vi "Move Left To Matrix.vi"(3 "Make Vertical":bool, 5 "Label":string="Test", 6 "Wait Time":dbl, 8 "error in":errorcluster, 9 "Speed (mm/s)":dbl=50.0, 10 "Offset":T1 format="%.3f", 11 "Location":string) -> (0 "error out":errorcluster)   [LabVIEW 2013]
uses:
  <vilib>/Analysis/Matrix/Datatypes/RealMatrix.ctl
  <vilib>/Analysis/Matrix/NI_Matrix.lvlib
panel:
  out "Final Offset":T1 format="%.3f"
  in  "Alt Goal":T2
  in  "Start":T1 format="%.3f"
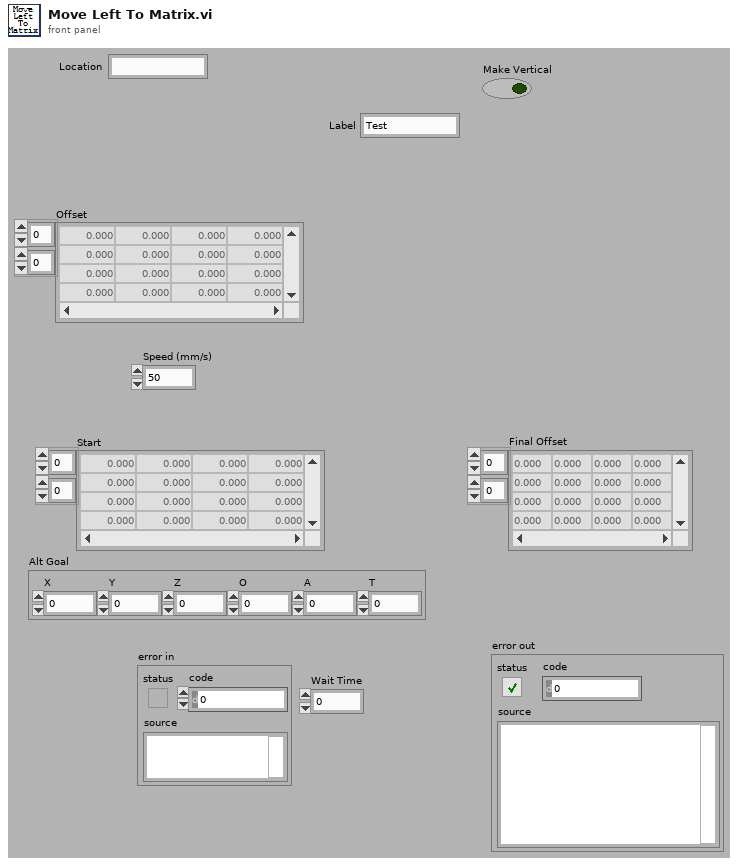
[diagram p1: front panel]
types:
  T1 = typedef "NI_Matrix.lvlib/RealMatrix.ctl" = dbl[][]
  T2 = cluster{"X":dbl, "Y":dbl, "Z":dbl, "O":dbl, "A":dbl, "T":dbl}
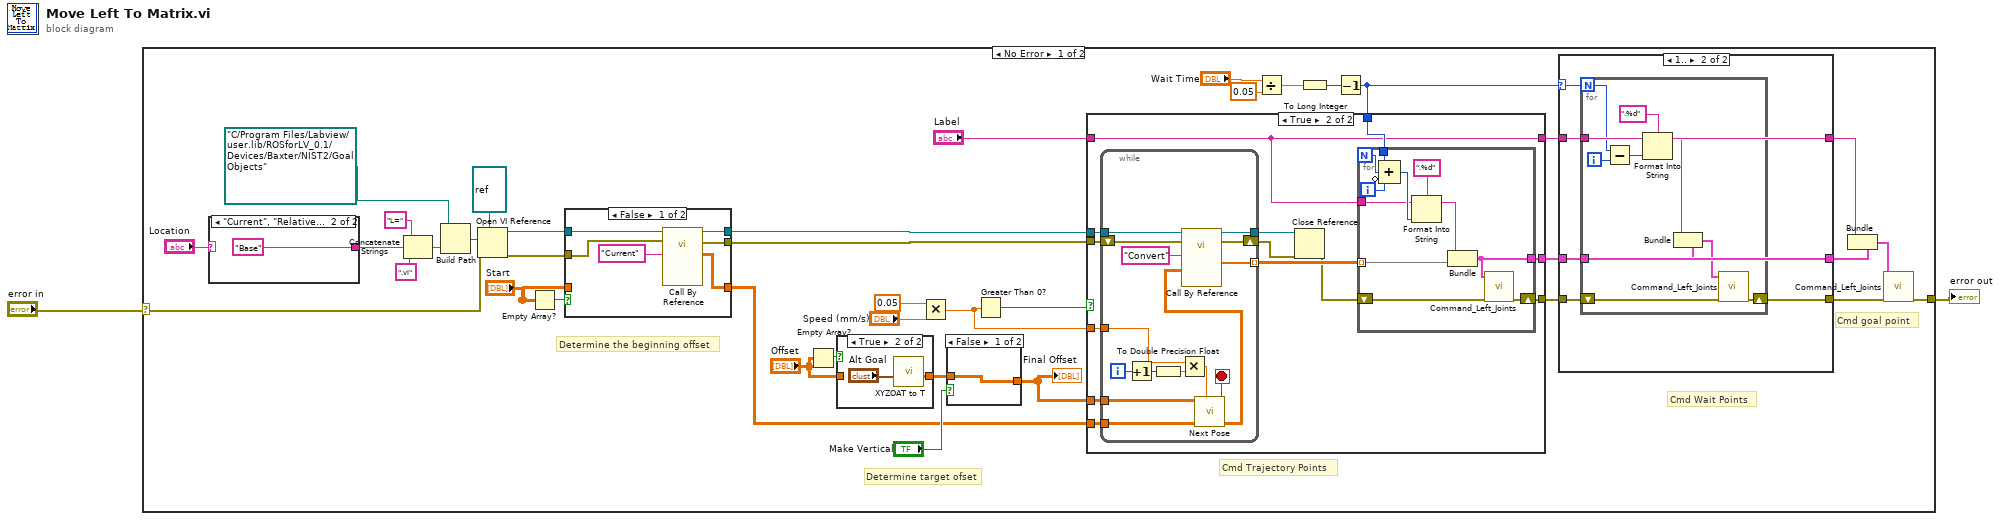
[diagram p0: block diagram]
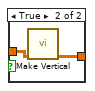
[diagram p5: hidden frame]
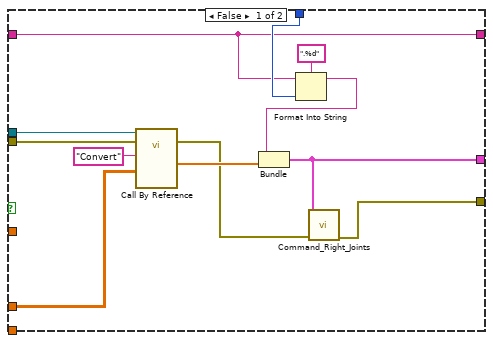
[diagram p6: hidden frame]
diagram:
  n1 = case shown="No Error" "error in" {
    selector: "error in" -> [w17 w128]
    tunnel: [w5 w128] -> w1
    frame No Error {
      # "Determine target ofset"
      # "Determine the beginning offset"
      # "Cmd goal point"
      # "Cmd Wait Points"
      # "Cmd Trajectory Points"
      n2 = case shown="\"Current\", \"Relative\"" "Location" {
        selector: "Location" -> [w51 _]
        tunnel: [w51 "Base"] -> w20
        frame Default {
        }
        frame "Current", "Relative" {
        }
      }
      n3 = Concatenate Strings("L=", w20, ".vi" ("string")) -> (w27:string)
      n4 = Build Path(base path=path "C:/Program Files/Labview/user.lib/ROSforLV_0.1/Devices/Baxter/NIST2/Goal Objects", name or relative path=w27) -> (appended path=w28:path)
      n5 = Open VI Reference(type specifier VI Refnum (for type only)=refnum<vi> refnum, vi path=w28, error in (no error)=w17) -> (vi reference=w25:refnum<vi>, error out=w26:errorcluster)  [unwired: 3 in]
      n6 = Empty Array?(array="Start") -> (empty?=w19:bool)
      n7 = case shown="False" w19 {
        tunnel: [w47 w48] -> w11
        tunnel: w26 -> [w46 w48]
        tunnel: [w45 w49] -> w12
        tunnel: w25 -> [w43 w49]
        tunnel: "Start" -> [_ w50]
        tunnel: [w42 w50] -> w16
        frame False {
          n8 = call-by-ref "?"(reference=w43, error in=w46, "Command"="Current") -> (reference out=w45:refnum<vi>, error out=w47:errorcluster, "Matrix"=w42:T1)  [unwired: 8 in, 2 out]
        }
        frame True {
        }
      }
      n9 = Empty Array?(array="Offset") -> (empty?=w41:bool)
      n10 = case shown="True" w41 {
        tunnel: "Offset" -> [w125 _]
        tunnel: [w125 w126] -> w37
        frame False {
        }
        frame True {
          n11 = call "XYZOAT to T.vi"("XYZOAT"="Alt Goal") -> ("T"=w126:T1)  [unwired: 10 in]
        }
      }
      n12 = Multiply(x=0.05 ("y"), y="Speed (mm/s)") -> (x*y=w13:dbl)
      n13 = case shown="False" "Make Vertical" {
        tunnel: w37 -> [w71 w73]
        tunnel: [w71 w72] -> w36
        frame False {
        }
        frame True {
          n14 = call "Make Vertical.vi"("Matrix"=w73) -> ("Vertical Matrix"=w72:T1)  [unwired: 10 in]
        }
      }
      "Final Offset" <- w36
      n15 = Greater Than 0?(x=w13) -> (x > 0?=w40:bool)
      n16 = Divide(x="Wait Time", y=0.05) -> (x/y=w31:dbl)
      n17 = To Long Integer(number=w31) -> (32bit integer=w30:i32)
      n18 = Decrement(x=w30) -> (x-1=w32:i32)
      n19 = case shown="True" w40 {
        tunnel: w16 -> [_ w98]
        tunnel: "Label" -> [w74 w89]
        tunnel: w36 -> [w82 w97]
        tunnel: w13 -> [_ w95]
        tunnel: w32 -> [w76 w96]
        tunnel: w12 -> [w84 w94]
        tunnel: w11 -> [w83 w93]
        tunnel: [w80 w91] -> w10
        tunnel: [w78 w90] -> w8
        tunnel: [w74 w89] -> w9
        frame False {
          n20 = call-by-ref "?"(reference=w84, error in=w83, "Matrix"=w82, "Command"="Convert") -> (error out=w79:errorcluster, "Joints"=w81:dbl[])  [unwired: 7 in, 3 out]
          n21 = Format Into String(format string=".%d", initial string=w74, w76) -> (resulting string=w75:string)  [unwired: 1 in, 1 out]
          n22 = Bundle(w75, "Joints"=w81) -> (w80:cluster{string, "Joints":dbl[]})  [unwired: 1 in]
          n23 = call "Command_Right_Joints.vi"("error in"=w79, "Goal"=w80) -> ("error out"=w78:errorcluster)  [unwired: 6 in, 1 out]
        }
        frame True {
          n24 = while {
            tunnel: w98 -> [w119]
            tunnel: w97 -> [w118]
            tunnel: w95 -> [w121]
            tunnel: w94 -> [w115]
            tunnel: [w112] -> w92 mode=indexing
            shift-right: [w111] -> w87
            shift-left: w93 -> [w114]
            tunnel: [w110] -> w88
            i -> [w123]
            stop <- w124 stop-if-true
            n25 = Increment(x=w123) -> (x+1=w117:i32)
            n26 = To Double Precision Float(number=w117) -> (double precision float=w122:dbl)
            n27 = Multiply(x=w121, y=w122) -> (x*y=w120:dbl)
            n28 = call "Next Pose.vi"("Step"=w120, "Start"=w119, "Goal"=w118) -> ("Pose"=w113:T1, "At Goal"=w124:bool)  [unwired: 7 in]
            n29 = call-by-ref "?"(reference=w115, error in=w114, "Matrix"=w113, "Command"="Convert") -> (reference out=w110:refnum<vi>, error out=w111:errorcluster, "Joints"=w112:dbl[])  [unwired: 7 in, 2 out]
          }
          n30 = Close Reference(reference=w88, error in (no error)=w87) -> (error out=w86:errorcluster)
          n31 = for {
            N -> [w109]
            tunnel: w89 -> [w105]
            tunnel: w96 -> [w104]
            tunnel: w92 -> [w102] mode=indexing
            shift-right: [w100] -> w90
            shift-left: w86 -> [w101]
            tunnel: [w99] -> w91
            i -> [w108]
            n32 = Compound Arithmetic op=ADD(w104, w109, invert w108) -> (w106:i32)
            n33 = Format Into String(format string=".%d", initial string=w105, w106) -> (resulting string=w103:string)  [unwired: 1 in, 1 out]
            n34 = Bundle(w103, "Joints"=w102) -> (w99:cluster{string, "Joints":dbl[]})  [unwired: 1 in]
            n35 = call "Command_Left_Joints.vi"("error in"=w101, "Goal"=w99) -> ("error out"=w100:errorcluster)  [unwired: 6 in, 1 out]
          }
        }
      }
      n36 = case shown="1.." w32 {
        selector: w32 -> [_ w60]
        tunnel: w10 -> [w54 w57]
        tunnel: w9 -> [w53 w56]
        tunnel: w8 -> [w55 w59]
        tunnel: [w55 w58] -> w4
        tunnel: [w54 w57] -> w7
        tunnel: [w53 w56] -> w6
        frame ..0 {
        }
        frame 1.. {
          n37 = for {
            N: w60 -> [w69]
            tunnel: w56 -> [w64]
            tunnel: w57 -> [w66]
            shift-right: [w63] -> w58
            shift-left: w59 -> [w62]
            i -> [w68]
            n38 = Subtract(x=w69, y=w68) -> (x-y=w70:i32)
            n39 = Format Into String(format string=".%d", initial string=w64, w70) -> (resulting string=w65:string)  [unwired: 1 in, 1 out]
            n40 = Bundle(cluster=w66, w65) -> (w61:cluster{string, "Joints":dbl[]})  [unwired: 1 in]
            n41 = call "Command_Left_Joints.vi"("error in"=w62, "Goal"=w61) -> ("error out"=w63:errorcluster)  [unwired: 6 in, 1 out]
          }
        }
      }
      n42 = Bundle(cluster=w7, w6) -> (w3:cluster{string, "Joints":dbl[]})  [unwired: 1 in]
      n43 = call "Command_Left_Joints.vi"("error in"=w4, "Goal"=w3) -> ("error out"=w5:errorcluster)  [unwired: 6 in, 1 out]
    }
    frame Error {
    }
  }
  "error out" <- w1
